vi "template.vi"() -> ()   [LabVIEW 2009]
uses:
  <vilib>/Utility/file.llb/Write To Spreadsheet File (DBL).vi
  <vilib>/Analysis/NI_AALBase.lvlib
panel:
  in  "Exit":bool
  out "Scanning":bool
  in  "Scan Save Path":path
  in  "Save Power Scan?":bool
  out "Power Scan":cluster{dbl[], dbl[]}(graph)
  in  "Abort\n Scan":bool
  in  "Wavelength\n   Step Size":dbl=1.0 min=0.1 max=100.0
  in  "Starting\nWavelength":dbl=400.0 min=400.0 max=2500.0
  in  "Ending\nWavelength":dbl=500.0 min=451.0 max=2501.0
  in  "Step Time (sec)":dbl=1.0 min=0.1 max=10.0 step=0.1
  in  "Measurement Save Path":path
  in  "Save Measurement?":bool
  out "Power Measurement":dbl[](graph)
  out "Readout value":dbl format="%^#_9e"
  out "Readout string":string
  in  "Timeout [ms]":i32=1000
  out "New":bool
  out "ZeroValue":dbl
  out "RANG_Val":dbl
  out "RANG_lbl":string
  out "Rng":string
  out "AUTO?":bool
  in  "AUTO":bool=TRUE
  in  "Range":i16=1 min=1 max=6 step=1
  out "PM Error log":string
  in  "Beam\nDiameter (mm)":dbl=4.0 min=1.0 max=9.0 step=0.5
  in  "BWIn":u16(ring) caption="Bandwidth" items=["HIGH", "LOW"]
  in  "Averaging Rate":i32=300 min=33 max=5000 step=1
  in  "Zero?":bool
  in  "Stop Measurement":bool
  out "IDN String":string
  out "Sensor SN":string
  out "Sensor Name":string
  out "Incrementing Down":bool
  out "Changing Wavelength":bool
  out "Incrementing Up":bool
  in  "Increment":dbl=10.0 min=0.1 max=50.0
  in  "Target\nWavelength":dbl=400.0 min=400.0 max=3000.0
  out "Wavelength (nm)":dbl
  out "Turning Turret":bool
  out "Current Blaze":string caption="Grating Blaze"
  out "Grating Density":dbl
  out "Grating Index":i32
  in  "Select Grating Blaze":string(combo)
  out "error out":errorcluster
  out "Status":string
  out "Emulating":bool
  out "Initialized":bool
  in  "Force\nInitialization":bool
  in  "Mono ID":string(combo)
  out "Current UniqueID":string
  in  "Measure Power":bool
  in  "Initialize":bool
  in  "Switch Turret":bool
  in  "Scan":bool
  in  "Increment Down":bool
  in  "Increment Up":bool
  in  "Change Wavelength":bool
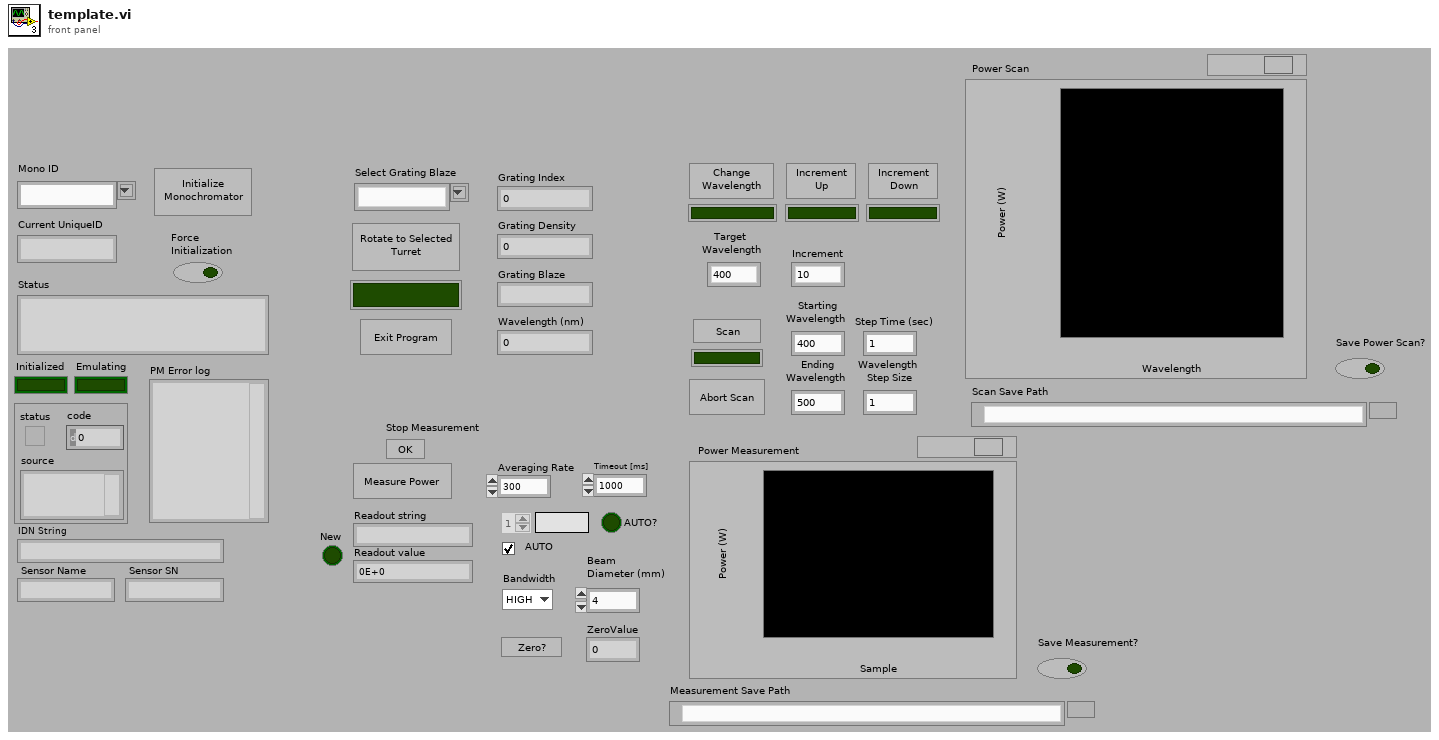
[diagram p1: front panel]
types:
  T1 = enum16{"0", "1", "2", "3", "4", "5", "6", "7", "8", "9"}
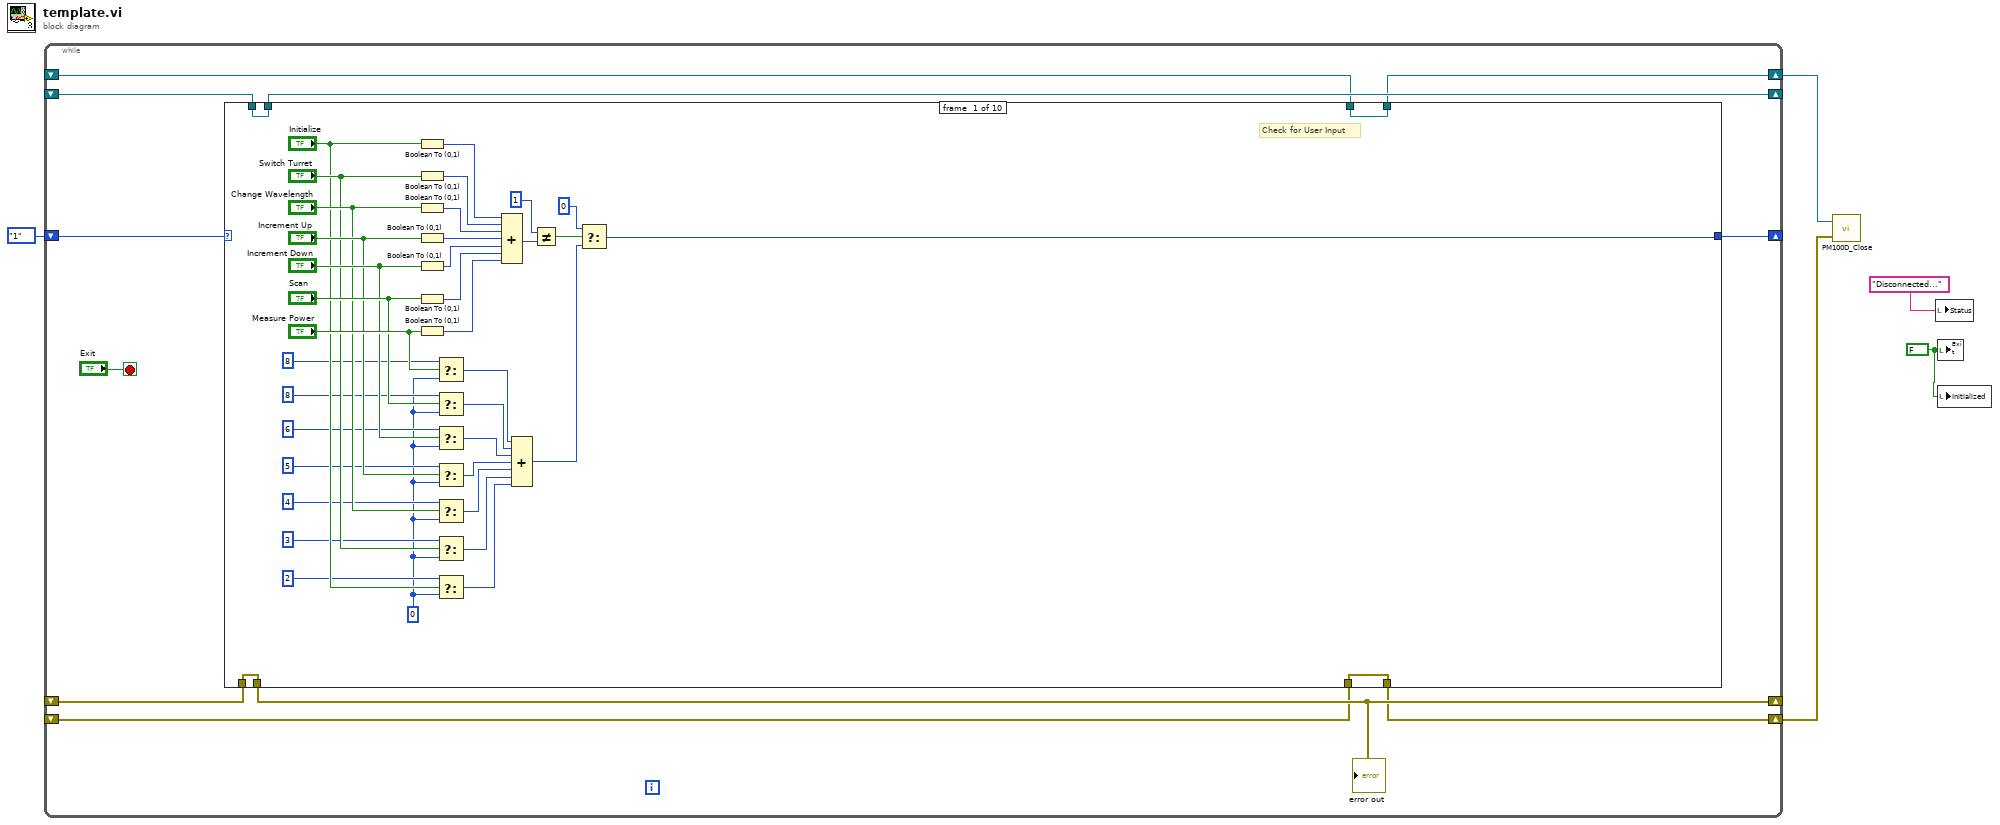
[diagram p0: block diagram]
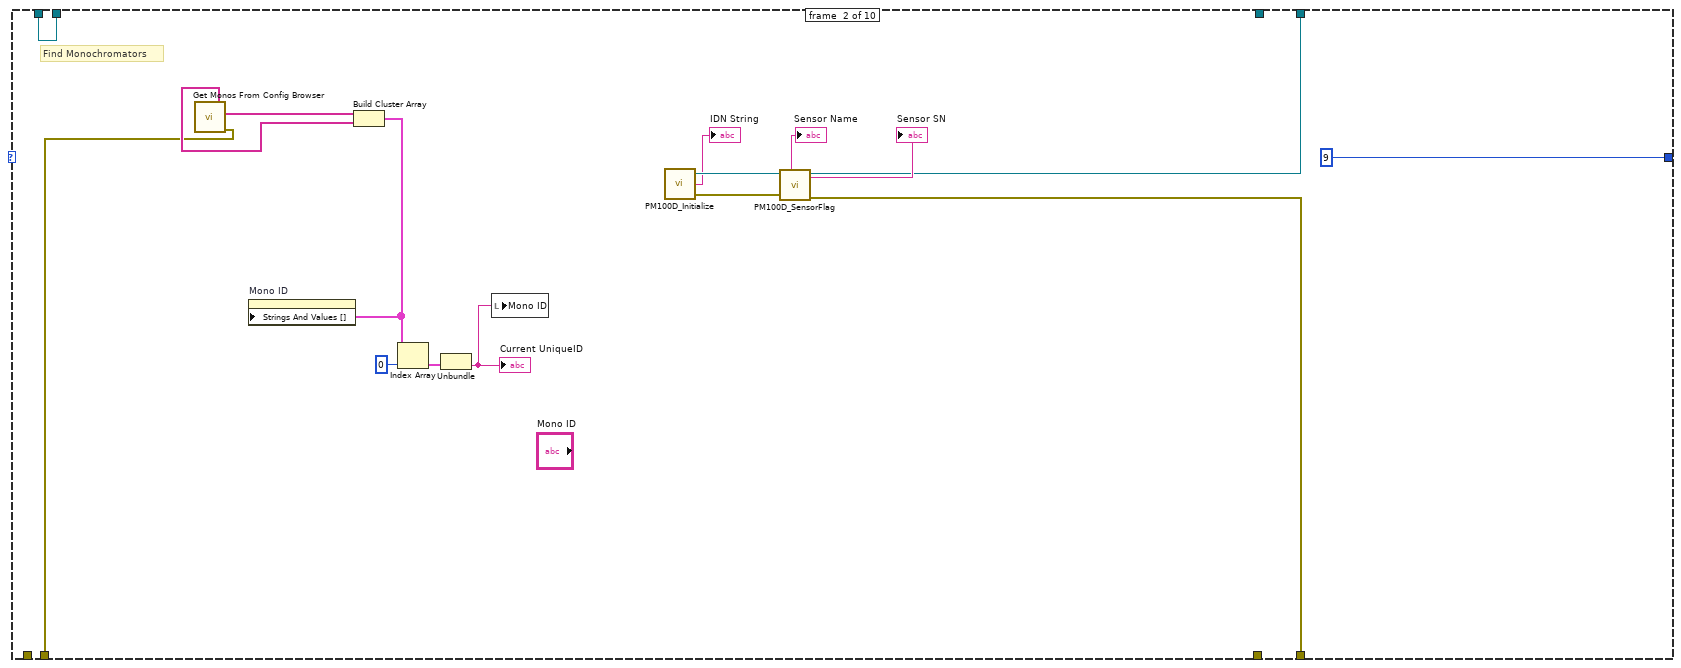
[diagram p2: hidden frame]
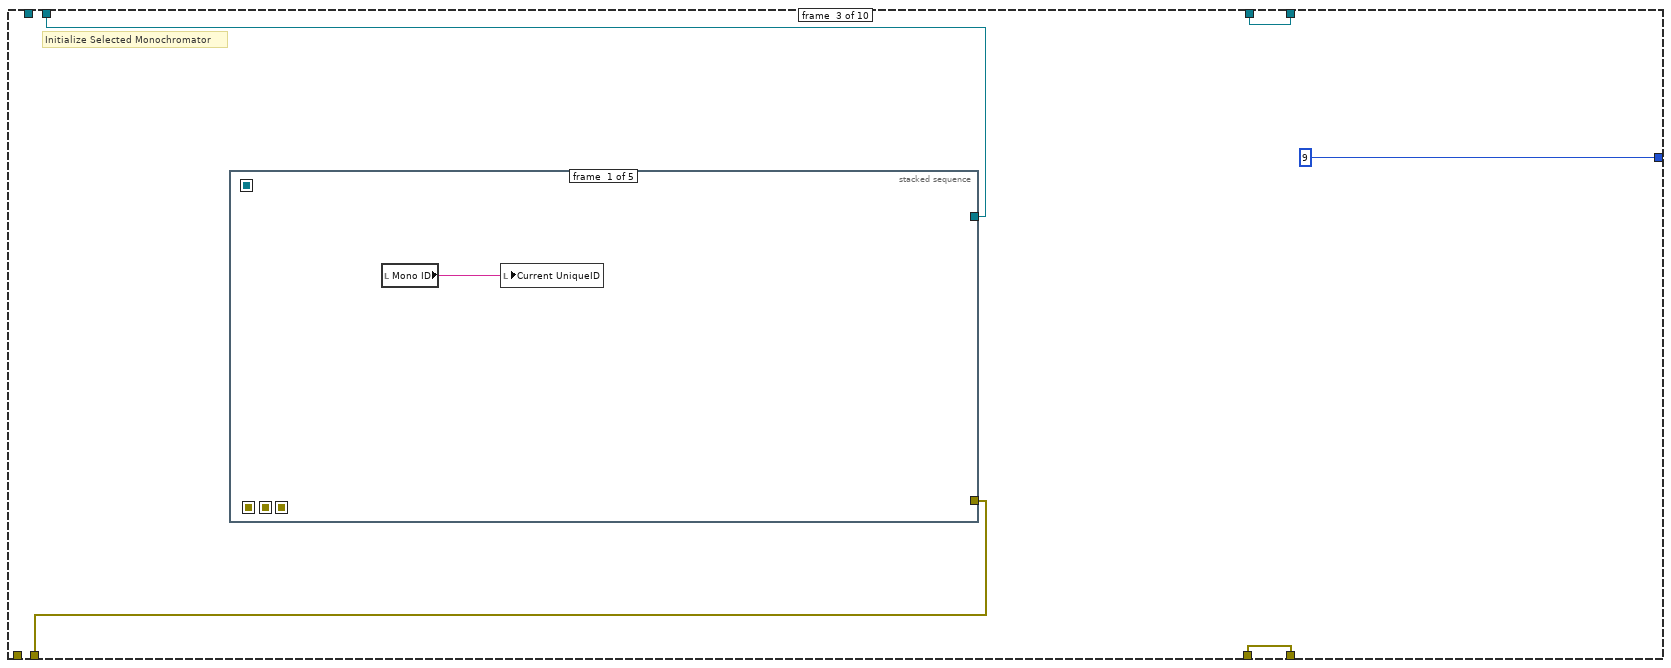
[diagram p3: hidden frame]
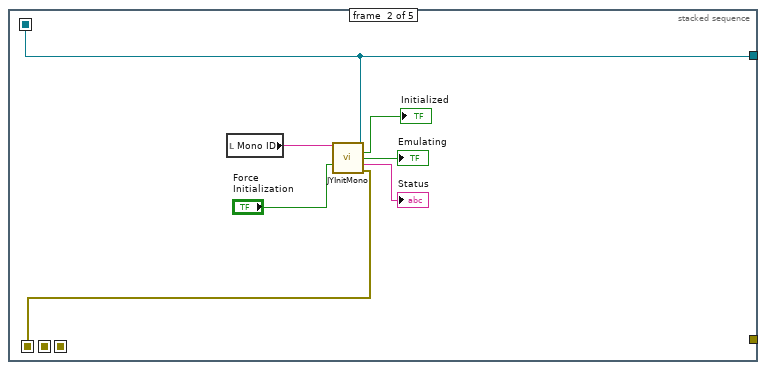
[diagram p4: hidden frame]
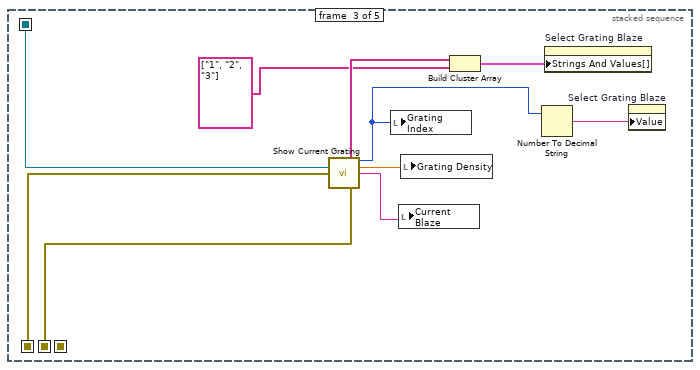
[diagram p5: hidden frame]
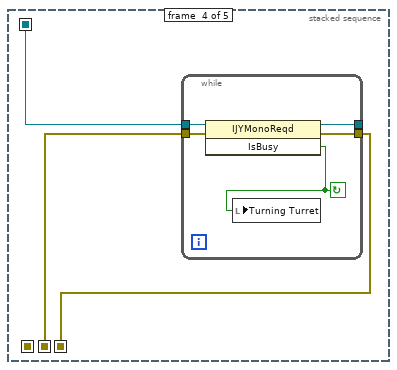
[diagram p6: hidden frame]
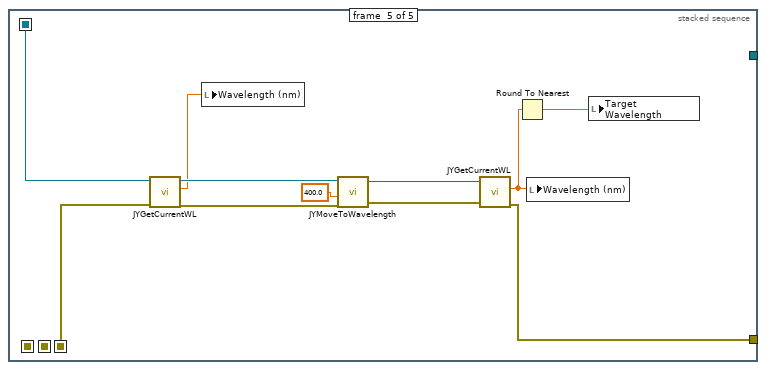
[diagram p7: hidden frame]
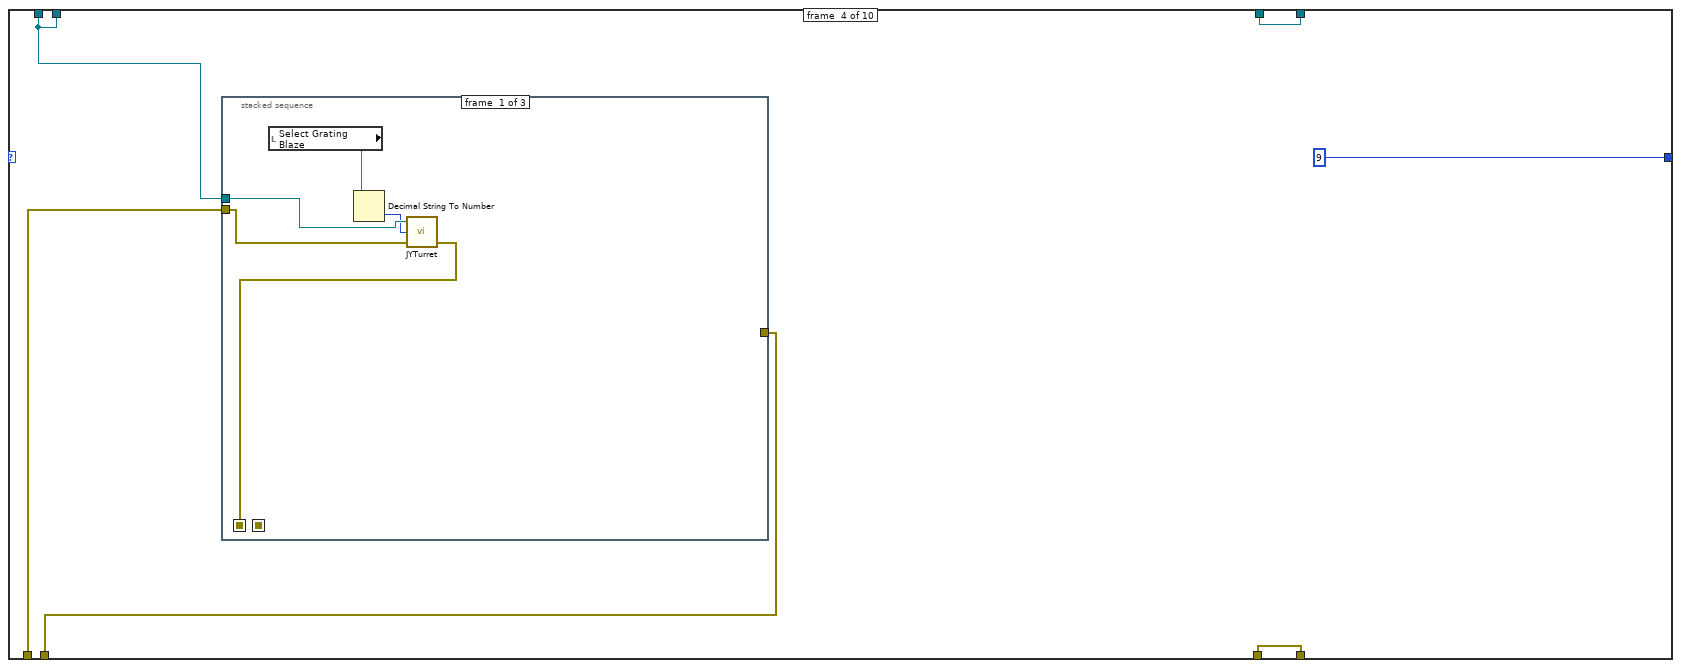
[diagram p8: hidden frame]
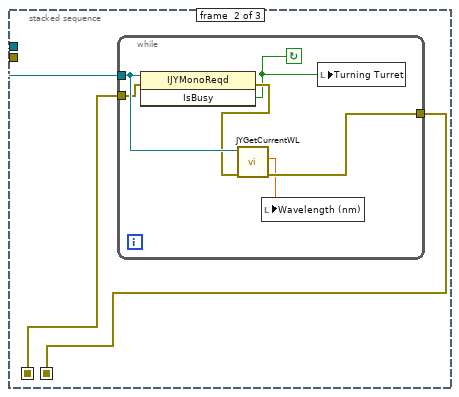
[diagram p9: hidden frame]
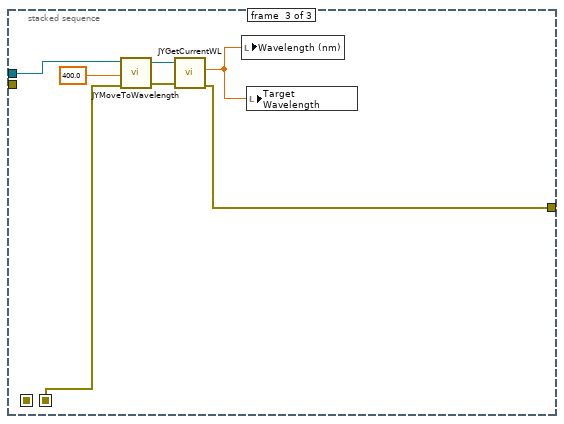
[diagram p10: hidden frame]
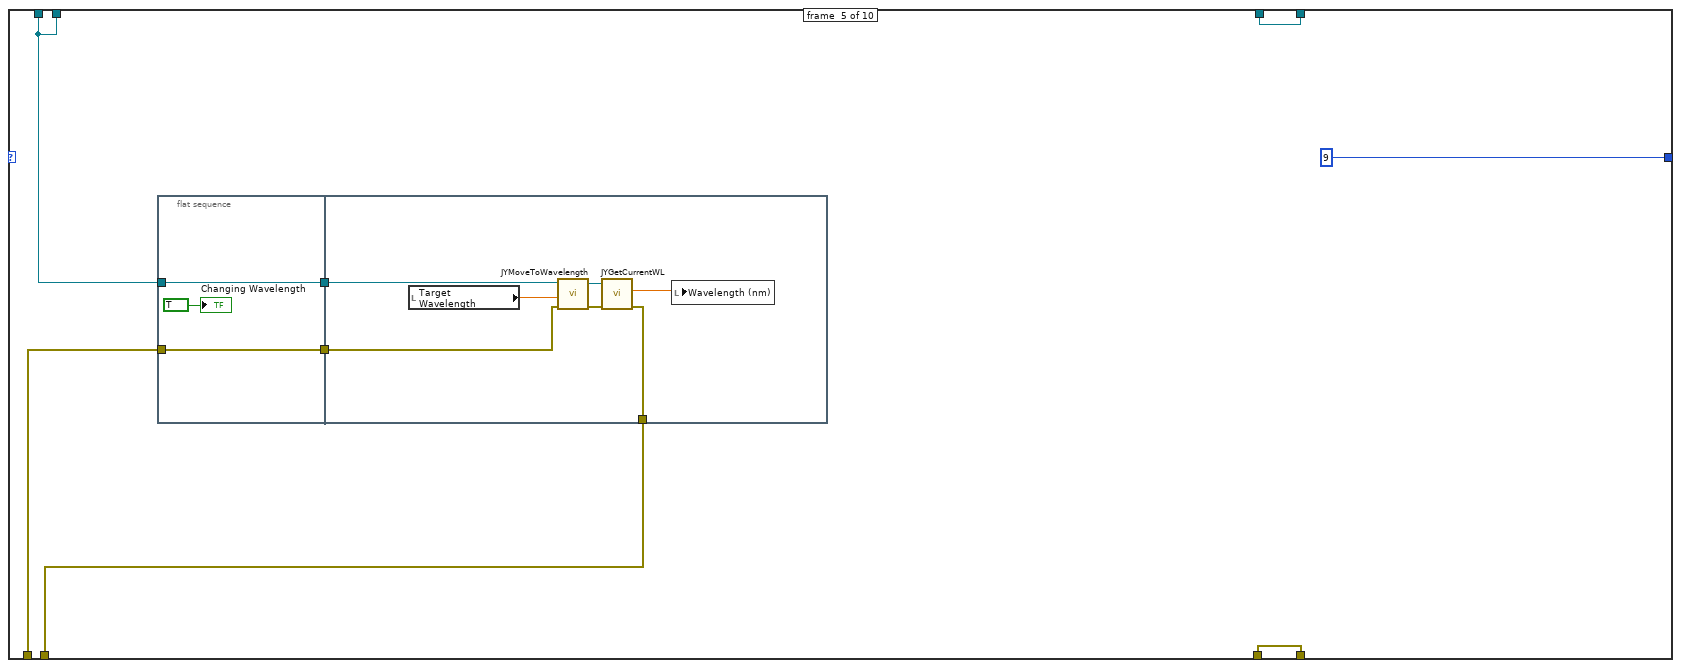
[diagram p11: hidden frame]
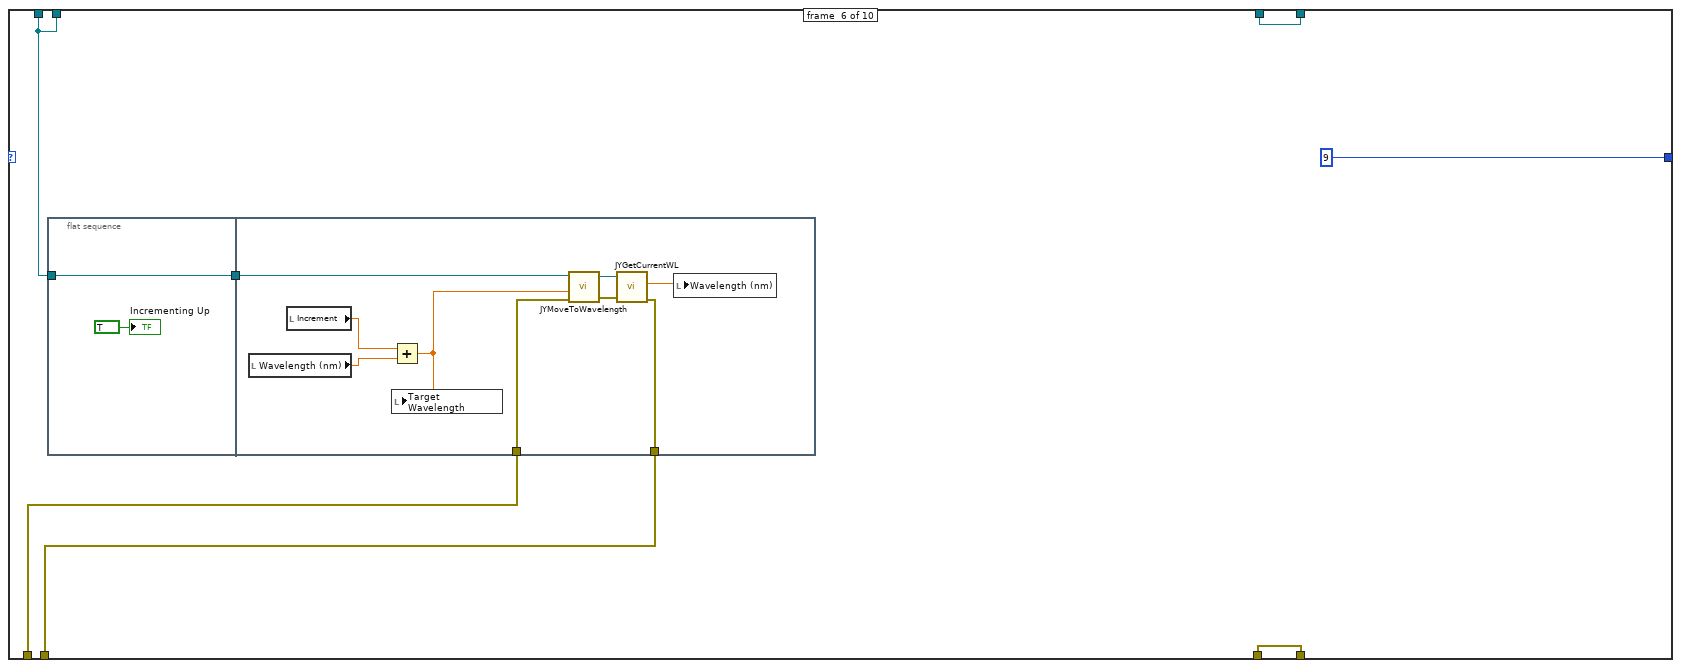
[diagram p12: hidden frame]
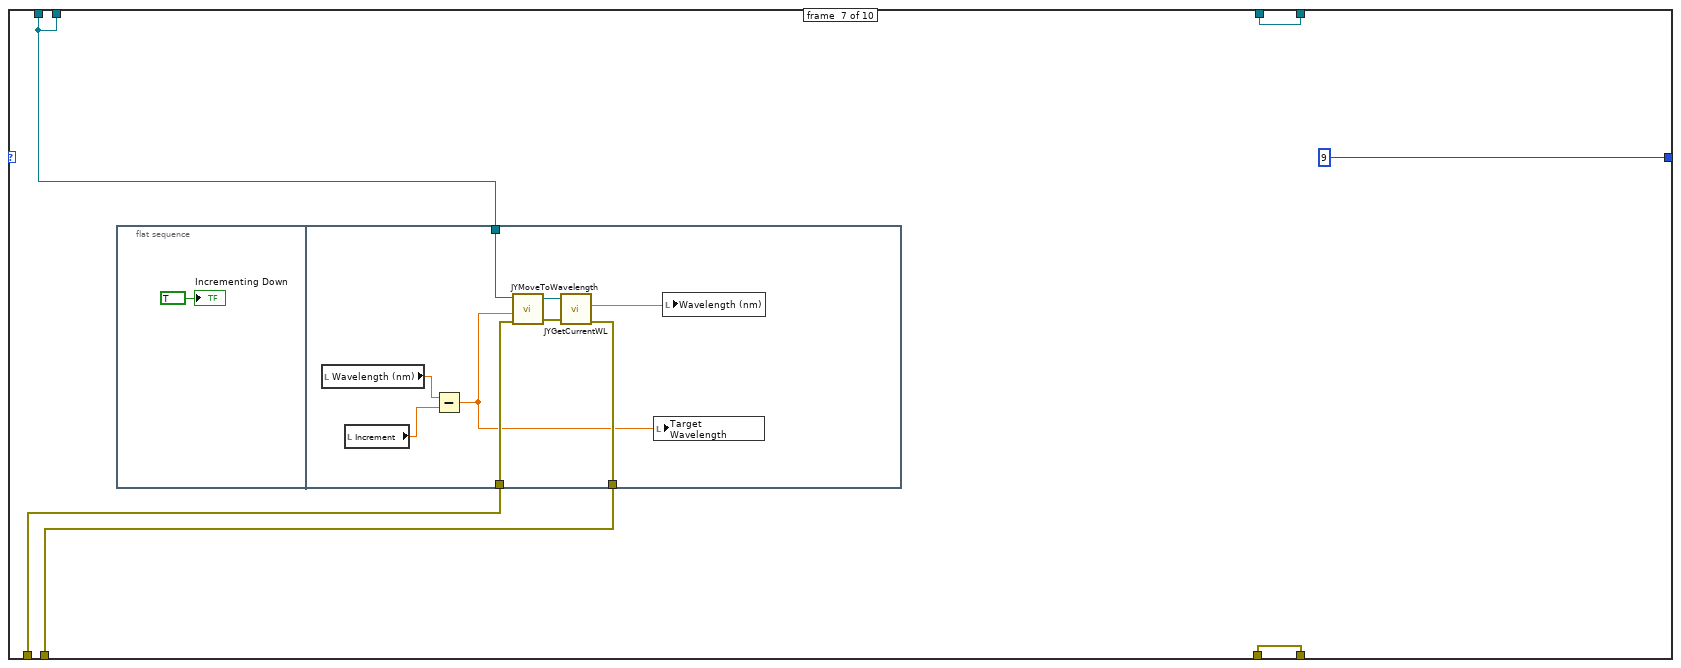
[diagram p13: hidden frame]
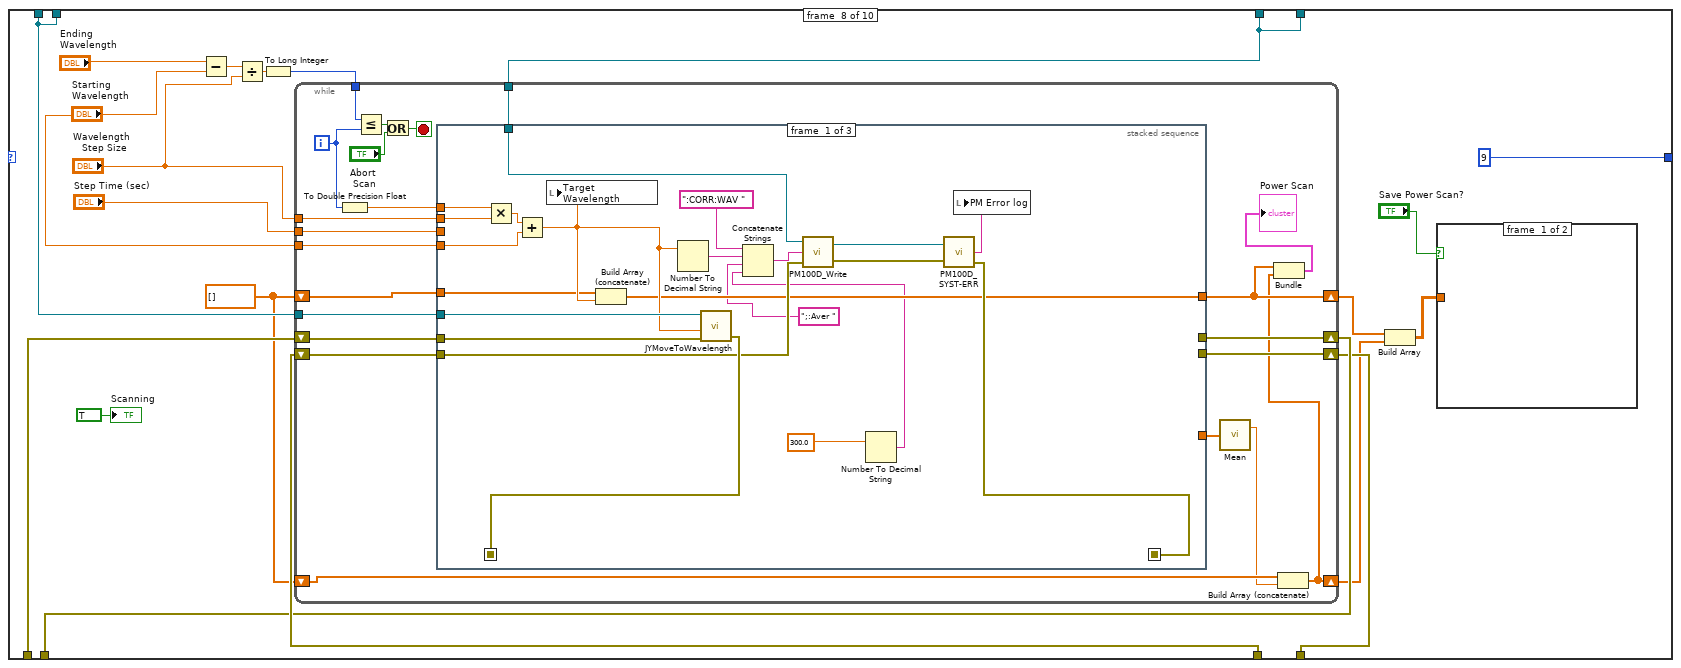
[diagram p14: hidden frame]
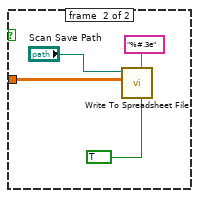
[diagram p15: hidden frame]
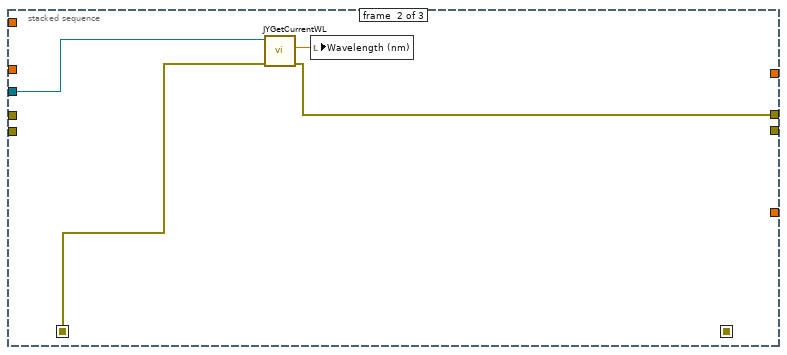
[diagram p16: hidden frame]
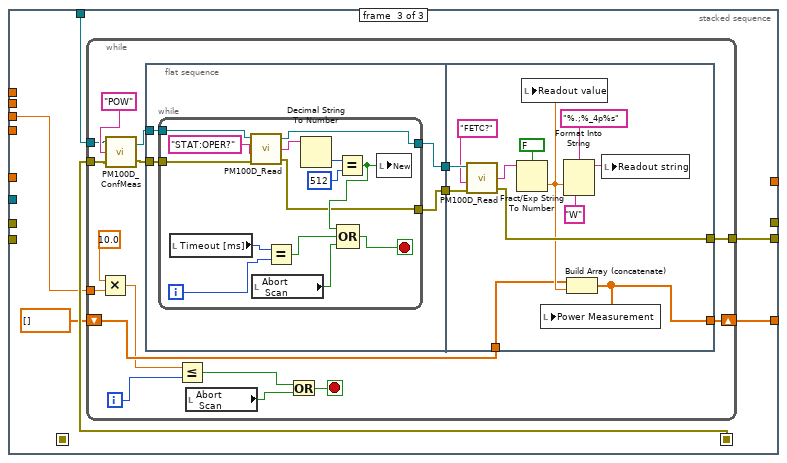
[diagram p17: hidden frame]
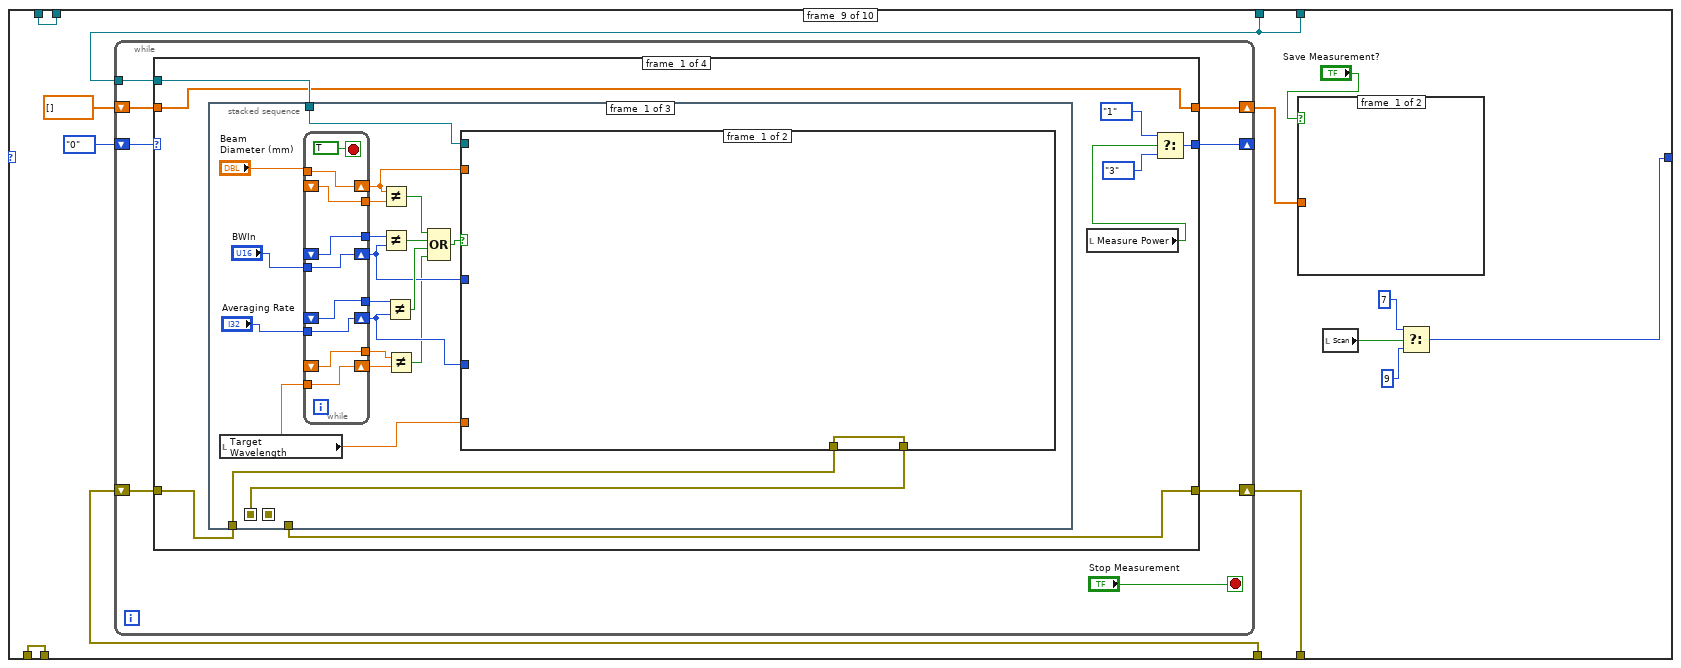
[diagram p18: hidden frame]
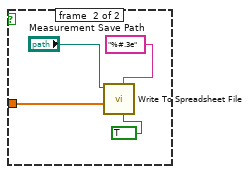
[diagram p19: hidden frame]
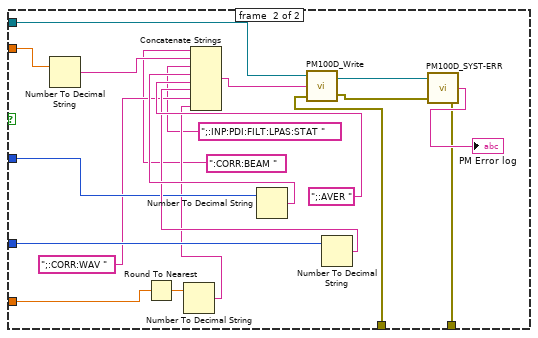
[diagram p20: hidden frame]
diagram:
  w1 = FALSE ("Exit")
  n1 = while {
    shift-right: [w16] -> _
    shift-left: T1."1" -> [w15]
    shift-right: [w14] -> _
    shift-left: _ -> [w13]
    shift-right: [w11] -> _
    shift-left: _ -> [w12]
    shift-right: [w10] -> w3
    shift-left: _ -> [w9]
    shift-right: [w8] -> w2
    shift-left: _ -> [w7]
    stop <- "Exit" stop-if-true
    n2 = case shown="7" w15 {
      tunnel: [w23 9 ("x") 9 ("x") 9 ("x") 9 ("x") 9 ("x") 9 ("x") 9 ("x") w318 0 ("x")] -> w16
      tunnel: [w20 w64 w75 w117 w146 w163 w179 w204 w329 w499] -> w14
      tunnel: [w19 w58 w74 w118 w145 w162 w181 w201 w330 w500] -> w11
      tunnel: w13 -> [w20 w64 _ w117 w146 w163 w179 w204 w329 w499]
      tunnel: w12 -> [w19 _ _ w116 w147 w164 w182 w203 w330 w500]
      tunnel: [w18 w57 w73 w115 w142 w160 w178 w200 w325 w497] -> w10
      tunnel: w9 -> [w18 _ w73 w115 w142 w160 w178 w202 w327 w497]
      tunnel: [w17 w56 w72 w114 w141 w159 w177 w194 w326 w498] -> w8
      tunnel: w7 -> [w17 _ w72 w114 w141 w159 w177 w194 w326 w498]
      frame #0 {
        w22 = 0 ("x")
        # "Check for User Input"
        n3 = Boolean To (0,1)(Boolean="Initialize") -> (0, 1=w55:i16)
        n4 = Boolean To (0,1)(Boolean="Switch Turret") -> (0, 1=w54:i16)
        n5 = Boolean To (0,1)(Boolean="Change Wavelength") -> (0, 1=w53:i16)
        n6 = Boolean To (0,1)(Boolean="Increment Up") -> (0, 1=w52:i16)
        n7 = Boolean To (0,1)(Boolean="Increment Down") -> (0, 1=w51:i16)
        n8 = Boolean To (0,1)(Boolean="Scan") -> (0, 1=w50:i16)
        n9 = Boolean To (0,1)(Boolean="Measure Power") -> (0, 1=w49:i16)
        n10 = Select(t=8 ("x"), s="Measure Power", f=w22) -> (s? t:f=w39:i32)
        n11 = Select(t=8 ("x"), s="Scan", f=w22) -> (s? t:f=w38:i32)
        n12 = Select(t=6 ("x"), s="Increment Down", f=w22) -> (s? t:f=w37:i32)
        n13 = Select(t=5 ("x"), s="Increment Up", f=w22) -> (s? t:f=w36:i32)
        n14 = Select(t=4 ("x"), s="Change Wavelength", f=w22) -> (s? t:f=w35:i32)
        n15 = Select(t=3 ("x"), s="Switch Turret", f=w22) -> (s? t:f=w34:i32)
        n16 = Select(t=2 ("x"), s="Initialize", f=w22) -> (s? t:f=w33:i32)
        n17 = Compound Arithmetic op=ADD(w55, w54, w53, w52, w51, w50, w49) -> (w48:i16)
        n18 = Compound Arithmetic op=ADD(w39, w38, w37, w36, w35, w34, w33) -> (w24:i32)
        n19 = Not Equal?(x=i16 1, y=w48) -> (x != y?=w32:bool)
        n20 = Select(t=0 ("x"), s=w32, f=w24) -> (s? t:f=w23:i32)
      }
      frame #1 {
        # "Find Monochromators"
        n21 = call "Get Monos From Config Browser.vi"() -> ("UniqueIDs"=w68:string[], "Mono ID"=w67:string[], "error out"=w58:errorcluster)  [unwired: 3 in]
        n22 = Build Cluster Array(w67, w68) -> (w70:cluster{"String":string, "String":string}[])
        n23 = property on="Mono ID" class="CmbBox"("Strings And Values []"=w70) -> ()  [unwired: 2 in, 2 out]
        n24 = Index Array(array=w70, index=0) -> (element=w69:cluster{"String":string, "String":string})
        n25 = Unbundle(w69) -> ("String"=w65:string)  [unwired: 1 out]
        "Current UniqueID" <- w65
        n26 = local write "Mono ID"(w65) -> ()
        n27 = call "PM100D_Initialize.vi"() -> ("error out"=w62:errorcluster, "Instrument"=→"IDN String":string, "VISA out"=w63:refnum<visa-resource-name>)  [unwired: 2 in, 1 out]
        n28 = call "PM100D_SensorFlag.vi"("error in (no error)"=w62, "VISA in"=w63) -> ("error out"=w57:errorcluster, "VISA out"=w56:refnum<visa-resource-name>, "sn"=→"Sensor SN":string, "name"=→"Sensor Name":string)  [unwired: 2 in, 4 out]
      }
      frame #2 {
        # "Initialize Selected Monochromator"
        n29 = stacked-sequence {
          seq-local: [_ w79 _ _ _] -> [_ _ w94 _ _]
          seq-local: [_ w78 _ _ _] -> [_ _ w93 w96 w111]
          seq-local: [_ _ w89 _ _] -> [_ _ _ w97 _]
          seq-local: [_ _ _ w95 _] -> [_ _ _ _ w112]
          tunnel: [_ _ _ _ w103] -> w74
          tunnel: [_ w78 _ _ _] -> w75
          frame #0 {
            n30 = local read "Mono ID"() -> (w77:string)
            n31 = local write "Current UniqueID"(w77) -> ()
          }
          frame #1 {
            n32 = local read "Mono ID"() -> (w80:string)
            n33 = call "JYInitMono.vi"("Unique ID"=w80, "Force Init"="Force\nInitialization") -> ("Mono RefNum out"=w78:refnum<k7>, "Initialized"=→"Initialized":bool, "Emulating"=→"Emulating":bool, "Status"=→"Status":string, "error out"=w79:errorcluster)  [unwired: 9 in]
          }
          frame #2 {
            n34 = call "Show Current Grating.vi"("Refnum in"=w93, "error in (no error)"=w94) -> ("Blazes"=w92:string[], "Grating Index"=w87:i32, "Current Grating"=w85:dbl, "Current Blaze"=w86:string, "error out"=w89:errorcluster)  [unwired: 5 in, 4 out]
            n35 = local write "Grating Index"(w87) -> ()
            n36 = local write "Current Blaze"(w86) -> ()
            n37 = local write "Grating Density"(w85) -> ()
            n38 = Build Cluster Array(w92, string[] ["1", "2", "3"]) -> (w90:cluster{"String":string, string}[])
            n39 = Number To Decimal String(number=w87) -> (decimal integer string=w88:string)  [unwired: 1 in]
            n40 = property on="Select Grating Blaze" class="CmbBox"("Strings And Values[]"=w90) -> ()  [unwired: 2 in, 2 out]
            n41 = property on="Select Grating Blaze" class="CmbBox"("Value"=w88) -> ()  [unwired: 2 in, 2 out]
          }
          frame #3 {
            n42 = while {
              tunnel: w96 -> [w102]
              tunnel: w97 -> [w101]
              tunnel: [w100] -> _
              tunnel: [w99] -> w95
              stop <- w98 continue-if-true
              n43 = invoke class="IJYMonoReqd" method="IsBusy"(reference=w102, error in=w101) -> (reference out=w100:refnum<k7>, error out=w99:errorcluster, "IsBusy"=w98:bool)  [unwired: 1 in]
              n44 = local write "Turning Turret"(w98) -> ()
            }
          }
          frame #4 {
            n45 = call "JYGetCurrentWL.vi"("error in (no error)"=w112, "JYMONOLib.IJYMonoReqd"=w111) -> ("error out"=w107:errorcluster, "Current WL"=w104:dbl, "Mono Refnum Out"=w110:refnum<k7>)  [unwired: 6 in, 1 out]
            n46 = local write "Wavelength (nm)"(w104) -> ()
            n47 = call "JYMoveToWavelength.vi"("error in (no error)"=w107, "Target WL"=400.0, "RefNum In"=w110) -> ("error out"=w106:errorcluster, "Refnum Out"=w109:refnum<k7>)  [unwired: 1 in, 1 out]
            n48 = call "JYGetCurrentWL.vi"("error in (no error)"=w106, "JYMONOLib.IJYMonoReqd"=w109) -> ("error out"=w103:errorcluster, "Current WL"=w105:dbl)  [unwired: 6 in, 2 out]
            n49 = Round To Nearest(number=w105) -> (nearest integer value=w108:dbl)
            n50 = local write "Wavelength (nm)"(w105) -> ()
            n51 = local write "Target\nWavelength"(w108) -> ()
          }
        }
      }
      frame #3 {
        n52 = stacked-sequence {
          seq-local: [w122 _ _] -> [_ w126 _]
          seq-local: [_ w125 _] -> [_ _ w135]
          tunnel: w116 -> [w124 _ _]
          tunnel: w117 -> [w123 w127 w139]
          tunnel: [_ _ w134] -> w118
          frame #0 {
            n53 = local read "Select Grating Blaze"() -> (w120:string)
            n54 = Decimal String To Number(string=w120) -> (number=w121:i32)  [unwired: 2 in, 1 out]
            n55 = call "JYTurret.vi"("error in (no error)"=w124, "Grating Index"=w121, "RefNum In"=w123) -> ("error out"=w122:errorcluster)  [unwired: 2 out]
          }
          frame #1 {
            n56 = while {
              tunnel: w127 -> [w133]
              tunnel: w126 -> [w132]
              tunnel: [w130] -> w125
              stop <- w129 continue-if-true
              n57 = invoke class="IJYMonoReqd" method="IsBusy"(reference=w133, error in=w132) -> (error out=w131:errorcluster, "IsBusy"=w129:bool)  [unwired: 1 in, 1 out]
              n58 = call "JYGetCurrentWL.vi"("error in (no error)"=w131, "JYMONOLib.IJYMonoReqd"=w133) -> ("error out"=w130:errorcluster, "Current WL"=w128:dbl)  [unwired: 6 in, 2 out]
              n59 = local write "Wavelength (nm)"(w128) -> ()
              n60 = local write "Turning Turret"(w129) -> ()
            }
          }
          frame #2 {
            n61 = call "JYMoveToWavelength.vi"("error in (no error)"=w135, "Target WL"=400.0, "RefNum In"=w139) -> ("error out"=w137:errorcluster, "Refnum Out"=w138:refnum<k7>)  [unwired: 1 in, 1 out]
            n62 = call "JYGetCurrentWL.vi"("error in (no error)"=w137, "JYMONOLib.IJYMonoReqd"=w138) -> ("error out"=w134:errorcluster, "Current WL"=w136:dbl)  [unwired: 6 in, 2 out]
            n63 = local write "Wavelength (nm)"(w136) -> ()
            n64 = local write "Target\nWavelength"(w136) -> ()
          }
        }
      }
      frame #4 {
        n65 = flat-sequence {
          tunnel: w146 -> [w150]
          tunnel: w147 -> [w151]
          tunnel: [w151] -> w144
          tunnel: [w150] -> w143
          tunnel: [w152] -> w145
          tunnel: w144 -> [w155]
          tunnel: w143 -> [w154]
          frame #0 {
            "Changing Wavelength" <- TRUE
          }
          frame #1 {
            n66 = local read "Target\nWavelength"() -> (w158:dbl)
            n67 = call "JYMoveToWavelength.vi"("error in (no error)"=w155, "Target WL"=w158, "RefNum In"=w154) -> ("error out"=w157:errorcluster, "Refnum Out"=w156:refnum<k7>)  [unwired: 1 in, 1 out]
            n68 = call "JYGetCurrentWL.vi"("error in (no error)"=w157, "JYMONOLib.IJYMonoReqd"=w156) -> ("error out"=w152:errorcluster, "Current WL"=w153:dbl)  [unwired: 6 in, 2 out]
            n69 = local write "Wavelength (nm)"(w153) -> ()
          }
        }
      }
      frame #5 {
        n70 = flat-sequence {
          tunnel: w163 -> [w167]
          tunnel: [w167] -> w161
          tunnel: w164 -> [w174]
          tunnel: [w170] -> w162
          tunnel: w161 -> [w171]
          frame #0 {
            "Incrementing Up" <- TRUE
          }
          frame #1 {
            n71 = local read "Wavelength (nm)"() -> (w175:dbl)
            n72 = local read "Increment"() -> (w176:dbl)
            n73 = Add(x=w176, y=w175) -> (x+y=w169:dbl)
            n74 = local write "Target\nWavelength"(w169) -> ()
            n75 = call "JYMoveToWavelength.vi"("error in (no error)"=w174, "Target WL"=w169, "RefNum In"=w171) -> ("error out"=w173:errorcluster, "Refnum Out"=w172:refnum<k7>)  [unwired: 1 in, 1 out]
            n76 = call "JYGetCurrentWL.vi"("error in (no error)"=w173, "JYMONOLib.IJYMonoReqd"=w172) -> ("error out"=w170:errorcluster, "Current WL"=w168:dbl)  [unwired: 6 in, 2 out]
            n77 = local write "Wavelength (nm)"(w168) -> ()
          }
        }
      }
      frame #6 {
        n78 = flat-sequence {
          tunnel: w182 -> [w188]
          tunnel: w179 -> [w187]
          tunnel: [w186] -> w181
          frame #0 {
            "Incrementing Down" <- TRUE
          }
          frame #1 {
            n79 = local read "Wavelength (nm)"() -> (w190:dbl)
            n80 = local read "Increment"() -> (w189:dbl)
            n81 = Subtract(x=w190, y=w189) -> (x-y=w185:dbl)
            n82 = call "JYMoveToWavelength.vi"("error in (no error)"=w188, "Target WL"=w185, "RefNum In"=w187) -> ("error out"=w192:errorcluster, "Refnum Out"=w191:refnum<k7>)  [unwired: 1 in, 1 out]
            n83 = call "JYGetCurrentWL.vi"("error in (no error)"=w192, "JYMONOLib.IJYMonoReqd"=w191) -> ("error out"=w186:errorcluster, "Current WL"=w184:dbl)  [unwired: 6 in, 2 out]
            n84 = local write "Target\nWavelength"(w185) -> ()
            n85 = local write "Wavelength (nm)"(w184) -> ()
          }
        }
      }
      frame #7 {
        w199 = dbl[] []
        n86 = Subtract(x="Ending\nWavelength", y="Starting\nWavelength") -> (x-y=w210:dbl)
        n87 = Divide(x=w210, y="Wavelength\n   Step Size") -> (x/y=w209:dbl)
        n88 = To Long Integer(number=w209) -> (32bit integer=w208:i32)
        n89 = while {
          tunnel: w208 -> [w238]
          tunnel: "Wavelength\n   Step Size" -> [w234]
          tunnel: "Step Time (sec)" -> [w233]
          tunnel: "Starting\nWavelength" -> [w232]
          tunnel: w204 -> [w229]
          shift-right: [w219] -> w198
          shift-left: w199 -> [w226]
          shift-right: [w225] -> w201
          shift-left: w203 -> [w228]
          tunnel: w194 -> [w224]
          shift-right: [w223] -> w200
          shift-left: w202 -> [w227]
          shift-right: [w218] -> w197
          shift-left: w199 -> [w221]
          i -> [w231]
          stop <- w236 stop-if-true
          n90 = To Double Precision Float(number=w231) -> (double precision float=w230:dbl)
          n91 = Less Or Equal?(x=w238, y=w231) -> (x <= y?=w237:bool)
          n92 = Or(x=w237, y="Abort\n Scan") -> (x .or. y?=w236:bool)
          n93 = stacked-sequence {
            seq-local: [w250 _ _] -> [_ w263 _]
            seq-local: [w248 _ _] -> [_ _ w270]
            tunnel: w234 -> [w256 _ _]
            tunnel: w233 -> [_ _ w266]
            tunnel: w232 -> [w253 _ _]
            tunnel: w230 -> [w255 _ _]
            tunnel: w229 -> [w252 w264 _]
            tunnel: w228 -> [w251 _ _]
            tunnel: w227 -> [w249 _ _]
            tunnel: w226 -> [w246 _ _]
            tunnel: [w245 _ _] -> w219
            tunnel: [_ w262 _] -> w225
            tunnel: w224 -> [w240 _ w269]
            tunnel: [_ _ w268] -> w223
            tunnel: [_ _ w265] -> w222
            frame #0 {
              n94 = Multiply(x=w255, y=w256) -> (x*y=w254:dbl)
              n95 = Add(x=w254, y=w253) -> (x+y=w247:dbl)
              n96 = local write "Target\nWavelength"(w247) -> ()
              n97 = Build Array (concatenate)(w246, w247) -> (w245:dbl[])
              n98 = Number To Decimal String(number=w247) -> (decimal integer string=w259:string)  [unwired: 1 in]
              n99 = call "JYMoveToWavelength.vi"("error in (no error)"=w251, "Target WL"=w247, "RefNum In"=w252) -> ("error out"=w250:errorcluster)  [unwired: 1 in, 2 out]
              n100 = Number To Decimal String(number=300.0 ("y")) -> (decimal integer string=w242:string)  [unwired: 1 in]
              n101 = Concatenate Strings(":CORR:WAV " ("string"), w259, ";:Aver " ("string"), w242) -> (w260:string)
              n102 = call "PM100D_Write.vi"("error in (no error)"=w249, "Command"=w260, "VISA in"=w240) -> ("error out"=w243:errorcluster, "VISA out"=w244:refnum<visa-resource-name>)
              n103 = call "PM100D_SYST-ERR.vi"("error out 2"=w243, "VISA In"=w244) -> ("error out"=w248:errorcluster, "Error"=w257:string)  [unwired: 1 in, 1 out]
              n104 = local write "PM Error log"(w257) -> ()
            }
            frame #1 {
              n105 = call "JYGetCurrentWL.vi"("error in (no error)"=w263, "JYMONOLib.IJYMonoReqd"=w264) -> ("error out"=w262:errorcluster, "Current WL"=w261:dbl)  [unwired: 6 in, 2 out]
              n106 = local write "Wavelength (nm)"(w261) -> ()
            }
            frame #2 {
              n107 = while {
                tunnel: w270 -> [w287]
                tunnel: w269 -> [w284]
                tunnel: [w280] -> w268
                shift-right: [w278] -> w265
                shift-left: dbl[] [] -> [w279]
                tunnel: w266 -> [w273]
                i -> [w274]
                stop <- w277 stop-if-true
                n108 = Multiply(x=10.0 ("y"), y=w273) -> (x*y=w271:dbl)
                n109 = call "PM100D_ConfMeas.vi"("error in"=w287, "Conf:"="POW" ("Command"), "VISA In"=w284) -> ("error out"=w286:errorcluster, "dup VISA session"=w283:refnum<visa-resource-name>)
                n110 = flat-sequence {
                  tunnel: w286 -> [w291]
                  tunnel: w283 -> [w290]
                  tunnel: [w289] -> w282
                  tunnel: [w288] -> w281
                  tunnel: w282 -> [w314]
                  tunnel: w281 -> [w313]
                  tunnel: [w309] -> w280
                  tunnel: w279 -> [w307]
                  tunnel: [w306] -> w278
                  frame #0 {
                    n111 = while {
                      tunnel: w291 -> [w295]
                      tunnel: [w294] -> w288
                      tunnel: w290 -> [w293]
                      tunnel: [w292] -> w289
                      i -> [w303]
                      stop <- w305 stop-if-true
                      n112 = local read "Timeout [ms]"() -> (w302:i32)
                      n113 = call "PM100D_Read.vi"("error in (no error)"=w295, "Command"="STAT:OPER?", "VISA in"=w293) -> ("error out"=w294:errorcluster, "ReadValue"=w297:string, "VISA out"=w292:refnum<visa-resource-name>)  [unwired: 1 in]
                      n114 = local read "Abort\n Scan"() -> (w304:bool)
                      n115 = Equal?(x=w302, y=w303) -> (x = y?=w301:bool)
                      n116 = Decimal String To Number(string=w297) -> (number=w300:i32)  [unwired: 2 in, 1 out]
                      n117 = Equal?(x=w300, y=512) -> (x = y?=w298:bool)
                      n118 = Compound Arithmetic op=OR(w298, w301, w304) -> (w305:bool)
                      n119 = local write "New"(w298) -> ()
                    }
                  }
                  frame #1 {
                    n120 = call "PM100D_Read.vi"("error in (no error)"=w313, "Command"="FETC?", "VISA in"=w314) -> ("error out"=w309:errorcluster, "ReadValue"=w311:string)  [unwired: 1 in, 1 out]
                    n121 = Fract/Exp String To Number(use system decimal point (T)=FALSE, string=w311) -> (number=w308:dbl)  [unwired: 2 in, 1 out]
                    n122 = local write "Readout value"(w308) -> ()
                    n123 = Format Into String(format string="%.;%_4p%s", w308, "W") -> (resulting string=w310:string)  [unwired: 2 in, 1 out]
                    n124 = Build Array (concatenate)(w307, w308) -> (w306:dbl[])
                    n125 = local write "Power Measurement"(w306) -> ()
                    n126 = local write "Readout string"(w310) -> ()
                  }
                }
                n127 = Less Or Equal?(x=w271, y=w274) -> (x <= y?=w276:bool)
                n128 = local read "Abort\n Scan"() -> (w275:bool)
                n129 = Or(x=w276, y=w275) -> (x .or. y?=w277:bool)
              }
            }
          }
          n130 = call <vilib>:"Mean.vi"("X"=w222) -> ("mean"=w220:dbl)  [unwired: 1 out]
          n131 = Build Array (concatenate)(w221, w220) -> (w218:dbl[])
          n132 = Bundle(w219, w218) -> (→"Power Scan":cluster{dbl[], dbl[]})  [unwired: 1 in]
        }
        n133 = Build Array(w198, w197) -> (w196:dbl[][])
        n134 = case shown="True" "Save Power Scan?" {
          tunnel: w196 -> [_ w213]
          frame #0 {
          }
          frame #1 {
            n135 = call-poly <vilib>:"Write To Spreadsheet File.vi"("transpose? (no:F)"=TRUE, "format (%.3f)"="%#.3e", "2D data"=w213, "file path (dialog if empty)"="Scan Save Path") -> ()  [unwired: 4 in, 1 out]
          }
        }
        "Scanning" <- TRUE ("Scanning")
      }
      frame #8 {
        n136 = while {
          shift-right: [w341] -> _
          shift-left: enum16{"0", "1", "2", "3"}."0" -> [w342]
          shift-right: [w338] -> w325
          shift-left: w327 -> [w340]
          tunnel: w326 -> [w339]
          shift-right: [w336] -> w322
          shift-left: dbl[] [] -> [w337]
          stop <- "Stop Measurement" stop-if-true
          n137 = case shown="\"0\", Default" w342 {
            tunnel: [w346 w463 enum16{"0", "1", "2", "3"}."0" enum16{"0", "1", "2", "3"}."0"] -> w341
            tunnel: w340 -> [w350 w461 w485 w494]
            tunnel: w339 -> [w349 w460 w486 _]
            tunnel: [w348 w458 w484 w494] -> w338
            tunnel: w337 -> [w347 w457 w481 w495]
            tunnel: [w347 w457 w480 w495] -> w336
            frame #0 {
              n138 = stacked-sequence {
                seq-local: [w357 _ _] -> [_ w403 _]
                seq-local: [_ w401 _] -> [_ _ w445]
                tunnel: w350 -> [w358 _ _]
                tunnel: w349 -> [w356 w402 w443]
                tunnel: [_ _ w444] -> w348
                frame #0 {
                  n139 = local read "Target\nWavelength"() -> (w351:dbl)
                  n140 = while {
                    shift-right: [w399] -> w359
                    shift-left: _ -> [w398]
                    shift-right: [w395] -> w360
                    shift-left: _ -> [w394]
                    shift-right: [w397] -> w355
                    shift-left: _ -> [w396]
                    tunnel: "Beam\nDiameter (mm)" -> [w399]
                    tunnel: [w398] -> w370
                    tunnel: "Averaging Rate" -> [w397]
                    tunnel: [w396] -> w369
                    tunnel: "BWIn" -> [w395]
                    tunnel: [w394] -> w361
                    shift-right: [w393] -> w353
                    shift-left: _ -> [w392]
                    tunnel: w351 -> [w393]
                    tunnel: [w392] -> w354
                    stop <- TRUE stop-if-true
                  }
                  n141 = Not Equal?(x=w359, y=w370) -> (x != y?=w366:bool)
                  n142 = Not Equal?(x=w361, y=w360) -> (x != y?=w367:bool)
                  n143 = Not Equal?(x=w369, y=w355) -> (x != y?=w368:bool)
                  n144 = Not Equal?(x=w354, y=w353) -> (x != y?=w352:bool)
                  n145 = Compound Arithmetic op=OR(w366, w367, w368, w352) -> (w365:bool)
                  n146 = case shown="True" w365 {
                    tunnel: w355 -> [_ w383]
                    tunnel: w360 -> [_ w382]
                    tunnel: w359 -> [_ w381]
                    tunnel: w358 -> [w371 w380]
                    tunnel: [w371 w379] -> w357
                    tunnel: w356 -> [_ w378]
                    tunnel: w351 -> [_ w374]
                    frame #0 {
                    }
                    frame #1 {
                      n147 = Number To Decimal String(number=w381) -> (decimal integer string=w384:string)  [unwired: 1 in]
                      n148 = Round To Nearest(number=w374) -> (nearest integer value=w377:dbl)
                      n149 = Number To Decimal String(number=w377) -> (decimal integer string=w375:string)  [unwired: 1 in]
                      n150 = Number To Decimal String(number=w382) -> (decimal integer string=w388:string)  [unwired: 1 in]
                      n151 = Number To Decimal String(number=w383) -> (decimal integer string=w385:string)  [unwired: 1 in]
                      n152 = Concatenate Strings(":CORR:BEAM " ("string"), w384, ";:INP:PDI:FILT:LPAS:STAT ", w388, ";:AVER " ("string"), w385, ";:CORR:WAV " ("string"), w375) -> (w391:string)
                      n153 = call "PM100D_Write.vi"("error in (no error)"=w380, "Command"=w391, "VISA in"=w378) -> ("error out"=w389:errorcluster, "VISA out"=w390:refnum<visa-resource-name>)
                      n154 = call "PM100D_SYST-ERR.vi"("error out 2"=w389, "VISA In"=w390) -> ("error out"=w379:errorcluster, "Error"=→"PM Error log":string)  [unwired: 1 in, 1 out]
                    }
                  }
                }
                frame #1 {
                  n155 = while {
                    shift-right: [w440] -> w404
                    shift-left: _ -> [w439]
                    shift-right: [w442] -> w405
                    shift-left: _ -> [w441]
                    tunnel: "AUTO" -> [w442]
                    tunnel: [w441] -> w411
                    tunnel: "Range" -> [w440]
                    tunnel: [w439] -> w408
                    stop <- TRUE stop-if-true
                  }
                  n156 = Not Equal?(x=w405, y=w411) -> (x != y?=w410:bool)
                  n157 = Not Equal?(x=w404, y=w408) -> (x != y?=w407:bool)
                  n158 = Or(x=w410, y=w407) -> (x .or. y?=w406:bool)
                  n159 = case shown="False" w406 {
                    tunnel: w405 -> [_ w420]
                    tunnel: w404 -> [_ w419]
                    tunnel: w402 -> [_ w417]
                    tunnel: [w413 w415] -> w401
                    tunnel: w403 -> [w413 w414]
                    frame #0 {
                    }
                    frame #1 {
                      n160 = Decrement(x=w419) -> (x-1=w427:i16)
                      n161 = call "PM100D_Ranging.vi"("VISA in"=w417, "Index"=w427, "AUTO"=w420, "error in (no error)"=w414, "Unit"="POW") -> ("SensType"=w426:i32, "AUTO?"=→"AUTO?":bool, "RANG_Val"=→"RANG_Val":dbl, "RANG_lbl"=w435:string, "error out"=w415:errorcluster)  [unwired: 3 in, 3 out]
                      "RANG_lbl" <- w435
                      n162 = Equal?(x=w426, y=1) -> (x = y?=w431:bool)
                      n163 = Equal?(x=w426, y=3) -> (x = y?=w421:bool)
                      n164 = Select(t=2, s=w420, f=0) -> (s? t:f=w433:i32)
                      n165 = Select(t=6, s=w431, f=4) -> (s? t:f=w432:i32)
                      n166 = Concatenate Strings(w435, "W") -> (→"Rng":string)
                      n167 = Not(x=w421) -> (.not. x?=w422:bool)
                      n168 = property on="Range" class="DigNum (strict)"("Disabled"=w433, "Maximum"=w432) -> ()  [unwired: 2 in, 2 out]
                      n169 = property on="AUTO" class="Bool (strict)"("Visible"=w422) -> ()  [unwired: 2 in, 2 out]
                    }
                  }
                }
                frame #2 {
                  n170 = case shown="False" "Zero?" {
                    tunnel: w443 -> [_ w454]
                    tunnel: w445 -> [w447 w452]
                    tunnel: [w447 w451] -> w444
                    tunnel: w443 -> [_ w450]
                    frame #0 {
                    }
                    frame #1 {
                      n171 = call "PM100D_Zeroing.vi"("VISA In"=w454) -> ("ZeroValue"=→"ZeroValue":dbl)  [unwired: 4 in]
                      n172 = call "PM100D_SYST-ERR.vi"("error out 2"=w452, "VISA In"=w450) -> ("error out"=w451:errorcluster, "Error"=w449:string)  [unwired: 1 in, 1 out]
                      n173 = local write "PM Error log"(w449) -> ()
                      n174 = local write "Zero?"(FALSE ("Zero?")) -> ()
                    }
                  }
                }
              }
              n175 = local read "Measure Power"() -> (w345:bool)
              n176 = Select(t=enum16{"0", "1", "2", "3"}."1", s=w345, f=enum16{"0", "1", "2", "3"}."3") -> (s? t:f=w346:enum16{"0", "1", "2", "3"})
            }
            frame #1 {
              n177 = call "PM100D_ConfMeas.vi"("error in"=w461, "Conf:"="POW" ("Command"), "VISA In"=w460) -> ("error out"=w459:errorcluster)  [unwired: 1 out]
              n178 = while {
                tunnel: w460 -> [w474]
                tunnel: w459 -> [w473]
                tunnel: [w472] -> _
                tunnel: [w471] -> w458
                tunnel: [w466] -> w462
                i -> [w468]
                stop <- w470 stop-if-true
                # "Query Operation Register for new data"
                n179 = Equal?(x="Timeout [ms]", y=w468) -> (x = y?=w467:bool)
                n180 = local read "Stop Measurement"() -> (w465:bool)
                n181 = call "PM100D_Read.vi"("error in (no error)"=w473, "Command"="STAT:OPER?", "VISA in"=w474) -> ("error out"=w471:errorcluster, "ReadValue"=w477:string, "VISA out"=w472:refnum<visa-resource-name>)  [unwired: 1 in]
                n182 = Decimal String To Number(string=w477) -> (number=w476:i32)  [unwired: 2 in, 1 out]
                n183 = Equal?(x=w476, y=512) -> (x = y?=w466:bool)
                "New" <- w466
                n184 = Compound Arithmetic op=OR(w466, w467, w465) -> (w470:bool)
              }
              n185 = Select(t=enum16{"0", "1", "2", "3"}."2", s=w462, f=enum16{"0", "1", "2", "3"}."1") -> (s? t:f=w463:enum16{"0", "1", "2", "3"})
            }
            frame #2 {
              n186 = call "PM100D_Read.vi"("error in (no error)"=w485, "Command"="FETC?", "VISA in"=w486) -> ("error out"=w484:errorcluster, "ReadValue"=w490:string)  [unwired: 1 in, 1 out]
              n187 = Fract/Exp String To Number(use system decimal point (T)=FALSE, string=w490) -> (number=w482:dbl)  [unwired: 2 in, 1 out]
              "Readout value" <- w482
              n188 = Build Array (concatenate)(w481, w482) -> (w480:dbl[])
              "Power Measurement" <- w480
              n189 = Format Into String(format string="%.;%_4p%s", w482, "W" ("Command")) -> (resulting string=→"Readout string":string)  [unwired: 2 in, 1 out]
            }
            frame #3 {
              n190 = local write "Stop Measurement"(TRUE ("t")) -> ()
            }
          }
        }
        n191 = case shown="False" "Save Measurement?" {
          tunnel: w322 -> [_ w331]
          frame #0 {
          }
          frame #1 {
            n192 = call-poly <vilib>:"Write To Spreadsheet File.vi"("transpose? (no:F)"=TRUE, "format (%.3f)"="%#.3e", "1D data"=w331, "file path (dialog if empty)"="Measurement Save Path") -> ()  [unwired: 4 in, 1 out]
          }
        }
        n193 = local read "Scan"() -> (w319:bool)
        n194 = Select(t=7 ("x"), s=w319, f=9 ("x")) -> (s? t:f=w318:i32)
      }
      frame #9 {
        w501 = FALSE
        n195 = local write "Stop Measurement"(w501) -> ()
        n196 = local write "Save Measurement?"(w501) -> ()
        n197 = local write "Abort\n Scan"(w501) -> ()
        n198 = local write "Save Power Scan?"(w501) -> ()
        n199 = local write "Incrementing Up"(w501) -> ()
        n200 = local write "Scanning"(w501) -> ()
        n201 = local write "Incrementing Down"(w501) -> ()
        n202 = local write "Changing Wavelength"(w501) -> ()
        n203 = local write "Initialize"(w501) -> ()
        n204 = local write "Switch Turret"(w501) -> ()
        n205 = local write "Change Wavelength"(w501) -> ()
        n206 = local write "Increment Up"(w501) -> ()
        n207 = local write "Increment Down"(w501) -> ()
        n208 = local write "Scan"(w501) -> ()
        n209 = local write "Measure Power"(w501) -> ()
        "Turning Turret" <- w501
      }
    }
    "error out" <- w11
  }
  n210 = call "PM100D_Close.vi"("error in (no error)"=w3, "VISA resource name"=w2) -> ()  [unwired: 2 in]
  n211 = local write "Status"("Disconnected...") -> ()
  n212 = local write "Exit"(w1) -> ()
  n213 = local write "Initialized"(w1) -> ()
